vi "Ausgabe_Diagramm.vi"(0 "Probenbezeichnung":string, 1 "Namen":string, 2 "Gruppe":string, 4 "Gewuenschte magn. Flussdichte [T]":dbl=0.001 min=0.001 max=5.0 step=0.001, 5 "Gwuenschte Frequenz [Hz]":dbl=15.0 min=15.0 max=15000.0 step=5.0, 6 "Eisenquerschnitt A [mm^2]":dbl=1.0 min=1.0 max=10000.0 step=1.0, 7 "Wirksame Laenge [cm]":dbl=94.0 min=0.0001 max=1000.0 step=0.5, 20 "Sekundaerwindungszahl":dbl=1.0 min=1.0 max=1500.0 step=1.0, 21 "Primaerwindungszahl":dbl=1.0 min=1.0 max=1500.0 step=1.0, 22 "Spannungsteilerverhaeltnis (1/x)":dbl=1.0 min=1.0 max=100.0 step=1.0, 23 "Dichte des Eisens in [g/cm^3]":dbl=1.0 min=1.0 max=50.0 step=1.0, 24 "Bmax [T]":dbl, 25 "Hmax [A/m]":dbl, 26 "Messwiderstand [Ohm]":dbl=1.0 min=1.0 max=100.0) -> ()   [LabVIEW 2016]
doc: "Plottet die Arrays für die Hystereseschleife und der Neukurve in einem XY-Graph.\n\nGibt die eingegebenen und berechnete Werte (Frequenz, Gruppe, etc.) aus.\n\nDas VI und der Graph können als PNG Datei abgespeichert werden."
panel:
  in  "Neukurve":dbl[][](array[numeric])=[[5.0, 1.0], [4.0, 4.0], [3.0, 6.0], [4.0, 3.0], [2.0, 6.0], [4.0, 4.0], [7.0, 4.0], [3.0, 5.0], [2.0, 6.0], [1.0, 7.0]]
  in  "Hystereseschleife":dbl[][](array[numeric])=[[0.0, 0.0], [1.0, 1.0], [2.0, 0.0], [3.0, 1.0], [4.0, 0.0], [-1.0, 1.0], [-2.0, 4.0], [-3.0, -5.0], [-4.0, 6.0], [-4.0, 7.0]]
  out "Namen":string
  out "Gruppe":string
  out "Probenbezeichnung":string
  out "Hmax [A/m]":dbl
  out "Bmax [T]":dbl
  out "Gwuenschte Frequenz [Hz]":dbl=15.0 min=15.0 max=15000.0 step=5.0
  out "Gewuenschte magn. Flussdichte [T]":dbl=0.001 min=0.001 max=5.0 step=0.001
  out "Messwiderstand [Ohm]":dbl=1.0 min=1.0 max=100.0
  out "Sekundaerwindungszahl":dbl=1.0 min=1.0 max=1500.0 step=1.0
  out "Primaerwindungszahl":dbl=1.0 min=1.0 max=1500.0 step=1.0
  out "Spannungsteilerverhaeltnis (1/x)":dbl=1.0 min=1.0 max=100.0 step=1.0
  out "Dichte des Eisens in [g/cm^3]":dbl=1.0 min=1.0 max=50.0 step=1.0
  out "Eisenquerschnitt A [mm^2]":dbl=1.0 min=1.0 max=10000.0 step=1.0
  out "Wirksame Laenge [cm]":dbl=94.0 min=0.0001 max=1000.0 step=0.5
  out "Hystereseschleife und Neukurve":cluster{dbl[], dbl[]}[](graph) caption="XY Graph"
  in  "Diagramm Speichern":bool
  in  "VI Speichern":bool
  out "Datum/Uhrzeit":timestamp
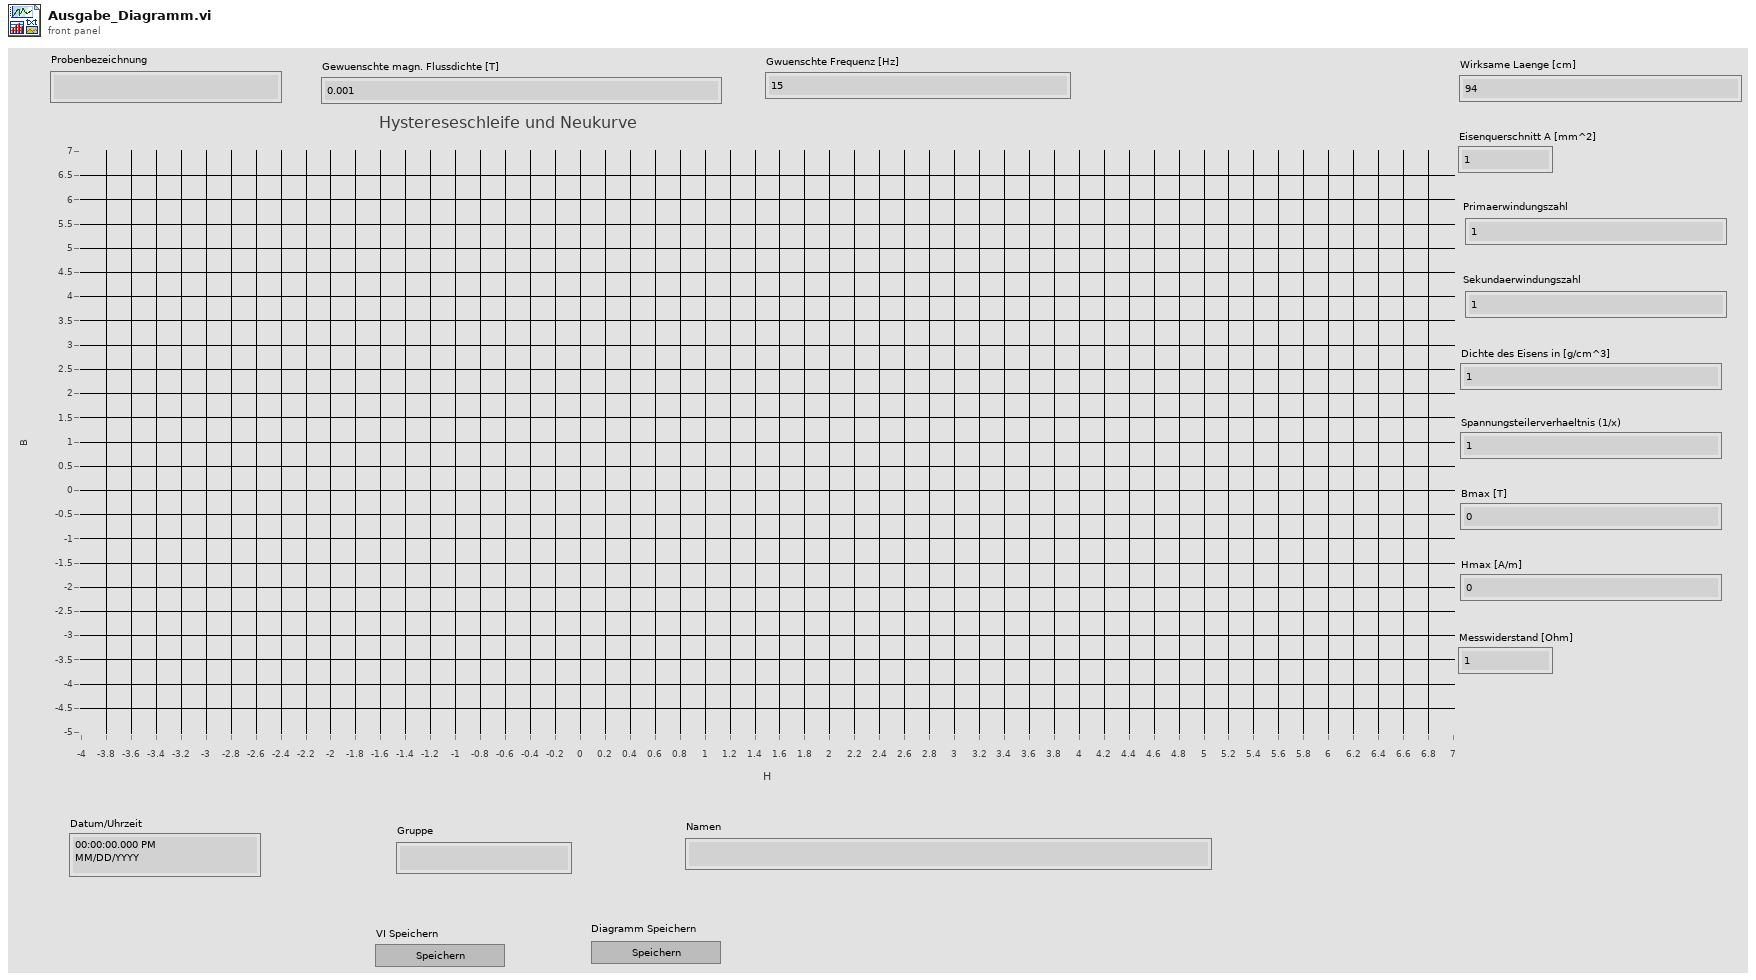
[diagram p1: front panel]
types:
  T1 = typedef "imagedata.ctl" = cluster{"image type":i32, "image depth":i32, "image":u8[], "mask":u8[], "colors":u32[], "Rectangle":cluster{"left":i16, "top":i16, "right":i16, "bottom":i16}}
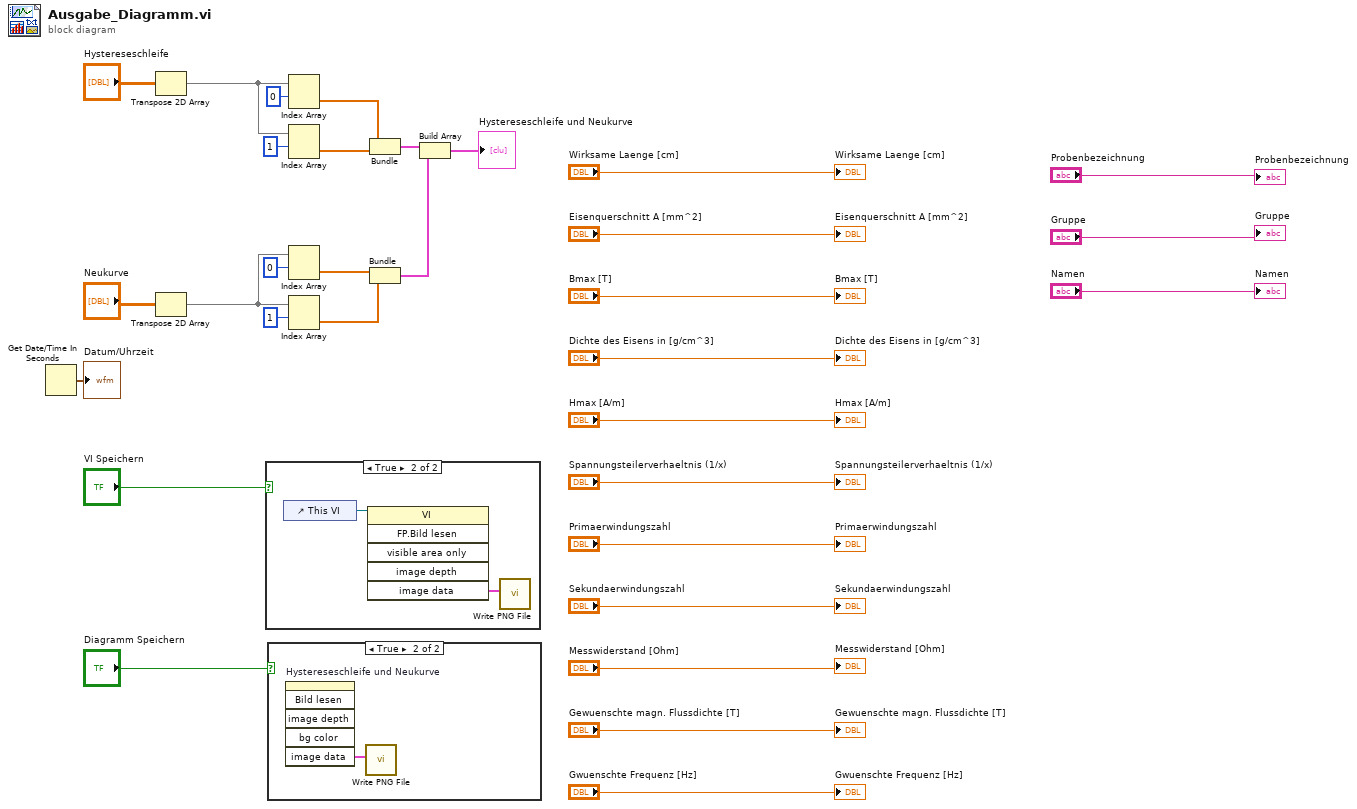
[diagram p0: block diagram]
diagram:
  n1 = Get Date/Time In Seconds() -> (seconds since 1Jan1904=→"Datum/Uhrzeit":timestamp)
  n2 = Transpose 2D Array(2D array="Hystereseschleife") -> (transposed array=w28:dbl[][])
  n3 = Transpose 2D Array(2D array="Neukurve") -> (transposed array=w18:dbl[][])
  n4 = case shown="True" "VI Speichern" {
    frame False {
    }
    frame True {
      n5 = control-ref of="This VI"() -> (w34:refnum<vi>)
      n6 = invoke class="VI" method="FP.Bild lesen"(reference=w34) -> ("image data"=w33:T1)  [unwired: 5 in, 5 out]
      n7 = call <vilib>:"Write PNG File.vi"("image data"=w33) -> ()  [unwired: 9 in, 2 out]
    }
  }
  n8 = case shown="True" "Diagramm Speichern" {
    frame False {
    }
    frame True {
      n9 = invoke on="Hystereseschleife und Neukurve" class="XYGraph (strikt)" method="Bild lesen"() -> ("image data"=w35:T1)  [unwired: 6 in, 5 out]
      n10 = call <vilib>:"Write PNG File.vi"("image data"=w35) -> ()  [unwired: 9 in, 2 out]
    }
  }
  n11 = Index Array(array=w28, index (row)=0) -> (element=w26:dbl[])  [unwired: 1 in]
  n12 = Index Array(array=w28, index (row)=1 ("Index (Zeile)")) -> (element=w25:dbl[])  [unwired: 1 in]
  n13 = Index Array(array=w18, index (row)=0) -> (element=w21:dbl[])  [unwired: 1 in]
  n14 = Index Array(array=w18, index (row)=1 ("Index (Zeile)")) -> (element=w20:dbl[])  [unwired: 1 in]
  n15 = Bundle(w26, w25) -> (w17:cluster{dbl[], dbl[]})  [unwired: 1 in]
  n16 = Bundle(w21, w20) -> (w19:cluster{dbl[], dbl[]})  [unwired: 1 in]
  n17 = Build Array(w17, w19) -> (→"Hystereseschleife und Neukurve":cluster{dbl[], dbl[]}[])
  "Wirksame Laenge [cm]" <- "Wirksame Laenge [cm]"
  "Eisenquerschnitt A [mm^2]" <- "Eisenquerschnitt A [mm^2]"
  "Dichte des Eisens in [g/cm^3]" <- "Dichte des Eisens in [g/cm^3]"
  "Spannungsteilerverhaeltnis (1/x)" <- "Spannungsteilerverhaeltnis (1/x)"
  "Primaerwindungszahl" <- "Primaerwindungszahl"
  "Sekundaerwindungszahl" <- "Sekundaerwindungszahl"
  "Messwiderstand [Ohm]" <- "Messwiderstand [Ohm]"
  "Gewuenschte magn. Flussdichte [T]" <- "Gewuenschte magn. Flussdichte [T]"
  "Gwuenschte Frequenz [Hz]" <- "Gwuenschte Frequenz [Hz]"
  "Bmax [T]" <- "Bmax [T]"
  "Hmax [A/m]" <- "Hmax [A/m]"
  "Probenbezeichnung" <- "Probenbezeichnung"
  "Gruppe" <- "Gruppe"
  "Namen" <- "Namen"
